vi "initialise.vi"(8 "error in (no error)":errorcluster, 11 "GenericPlugin in":refnum<class "FPGAWrapperRK110512Fiber_Spiral.lvclass">) -> (0 "error out":errorcluster, 3 "GenericPlugin out":refnum<class "FPGAWrapperRK110512Fiber_Spiral.lvclass">)   [LabVIEW 2010, in "FPGAWrapperRK110512Fiber_Spiral.lvclass"]
doc: "The dynamic dispatch-version of this VI initalises the plug-in object by allocating and initalising any dynamic resources need."
uses:
  FPGAWrapperRK110512Fiber_Spiral.lvclass
  GenericFPGAWrapper/GenericFPGAWrapper/GenericFPGAWrapper.lvclass
  <vilib>/rvi/interface/nirviOpenFPGA/nirviOpenFPGA.xnode
  config_data_cluster.ctl
  <vilib>/userDefined/High Color/nirio_resource_hc.ctl
  <vilib>/rvi/interface/nirviMethod/nirviMethod.xnode
  <vilib>/FPGAPlugInAG/Dynamic/niLvFpga_Reset_Dynamic.vi
  <vilib>/rvi/interface/nirviReadWriteControl/nirviReadWriteControl.xnode
  NiFpgaLv.dll
  <vilib>/Utility/error.llb/Error Cluster From Error Code.vi
  <vilib>/rvi/errors/niLvFpgaWhatHappensToTopLevelVI.ctl
  <vilib>/rvi/interface/common/niFpgaNodeNameForErrorReporting.ctl
  <vilib>/rvi/errors/niLvFpgaAdjustHostInterfaceError.vi
  FPGA_VI_Reference.ctl
  FPGA Bitfiles/FPGAWrapperRK120_FPGATarget_FPGASpiral_DEAF4785.lvbitx
  <vilib>/FPGAPlugInAG/PXI-7813R/niLvFpga_Open_PXI-7813R.vi
  <vilib>/rvi/ClientSDK/nirviWhatTheDeviceIsDoing.ctl
  <vilib>/rvi/interface/common/dynamic/niFpgaDynamicAddResources.vi
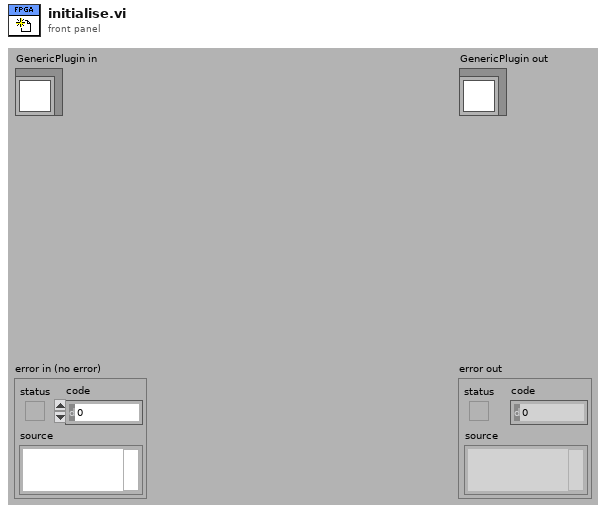
[diagram p1: front panel]
types:
  T1 = typedef "FPGAWrapperRK110512Fiber_Spiral.lvclass/FPGA_VI_Reference.ctl" = refnum<k20>
  T2 = typedef "nirio_resource_hc.ctl" = tag
  T3 = typedef "FPGAWrapperRK110512Fiber_Spiral.lvclass/config_data_cluster.ctl" = cluster{"Hifo box version":i16, "ADC clock phase":u8, "Enable ADC clock":bool, "FPGA Clock":u32}
  T4 = typedef "niFpgaNodeNameForErrorReporting.ctl" = enum16{"Open FPGA VI Reference", "Read/Write Control", "Invoke Method: Abort", "Invoke Method: Acknowledge IRQ", "Invoke Method: Download", "Invoke Method: FIFO.Configure", "Invoke Method: FIFO.Read", "Invoke Method: FIFO.Start", "Invoke Method: FIFO.Stop", "Invoke Method: FIFO.Write", "Invoke Method: Reset", "Invoke Method: Run", "Invoke Method: Wait on IRQ", "Close FPGA VI Reference"}
  T5 = typedef "niLvFpgaWhatHappensToTopLevelVI.ctl" = enum16{"top level VI scripted behind XNode", "top level VI inlined behind XNode"}
  T6 = typedef "nirviWhatTheDeviceIsDoing.ctl" = enum32{"nothing", "something other than LabVIEW FPGA", "FPGA interface", "interactive", "emulation"}
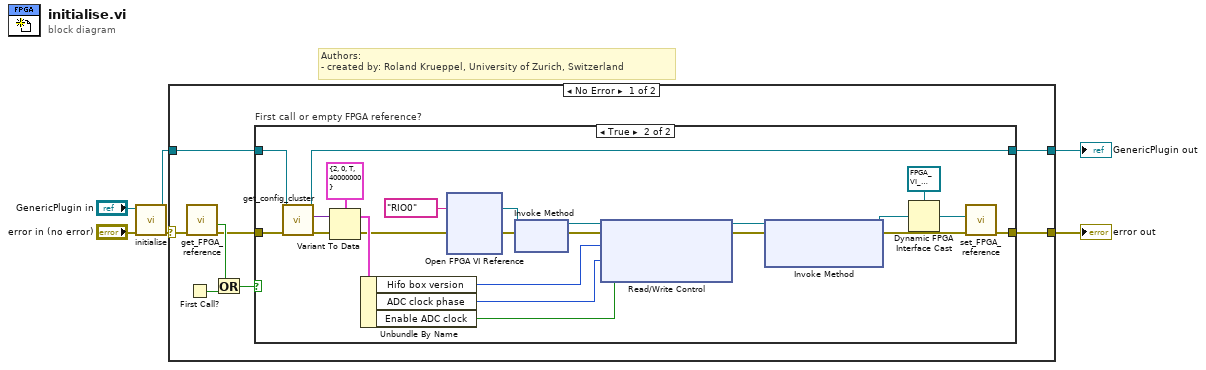
[diagram p0: block diagram]
diagram:
  # "Authors: \n- created by: Roland Krueppel, University of Zurich, Switzerland"
  n1 = call-parent "initialise.vi"("error in (no error)"="error in (no error)", "GenericPlugin in"="GenericPlugin in") -> ("error out"=w4:errorcluster, "GenericPlugin out"=w2:refnum<class "FPGAWrapperRK110512Fiber_Spiral.lvclass">)  [unwired: 8 in]
  n2 = case shown="No Error" w4 {
    selector: w4 -> [w14 w221]
    tunnel: [w7 w221] -> w3
    tunnel: [w10 w222] -> w1
    tunnel: w2 -> [w8 w222]
    frame No Error {
      n3 = First Call?() -> (First Call?: T/F=w13:bool)
      n4 = call "get_FPGA_reference.vi"("error in (no error)"=w14) -> ("error out"=w9:errorcluster, "is empty?"=w12:bool)  [unwired: 8 in, 1 out]
      n5 = Or(x=w12, y=w13) -> (x .or. y?=w11:bool)
      n6 = case "First call or empty FPGA reference?" shown="True" w11 {
        tunnel: [w15 w20] -> w10
        tunnel: w9 -> [w16 w39]
        tunnel: [w16 w22] -> w7
        tunnel: w8 -> [w15 w21]
        frame False {
        }
        frame True {
          n7 = call-dynamic "get_config_cluster.vi"("error in (no error)"=w39, "FPGAWrapperRK120511Fiber_Spiral in"=w21) -> ("error out"=w38:errorcluster, "config cluster (variant)"=w37:variant, "FPGAWrapperRK120511Fiber_Spiral out"=w20:refnum<class "FPGAWrapperRK110512Fiber_Spiral.lvclass">)  [unwired: 7 in]
          n8 = Variant To Data(error in=w38, Variant=w37, type=T3 {"Hifo box version"=2, "ADC clock phase"=0, "Enable ADC clock"=TRUE, "FPGA Clock"=40000000} ("config data")) -> (error out=w34:errorcluster, data=w35:T3)
          n9 = Unbundle By Name(w35) -> ("Hifo box version"=w28:i16, "ADC clock phase"=w27:u8, "Enable ADC clock"=w26:bool)
          n10 = xnode "Open FPGA VI Reference"("error in"=w34, "resource name"=T2 "RIO0") -> ("FPGA VI Reference Out"=w31:refnum<k20>, "error out"=w32:errorcluster)
          n11 = xnode "Invoke Method"("FPGA VI Reference In"=w31, "error in"=w32) -> ("FPGA VI Reference Out"=w29:refnum<k20>, "error out"=w30:errorcluster)
          n12 = xnode "Read/Write Control"("FPGA VI Reference In"=w29, "error in"=w30, "converter box version"=w28, "ADC clock phase"=w27, "Enable ADC clock?"=w26) -> ("FPGA VI Reference Out"=w25:refnum<k20>, "error out"=w24:errorcluster)
          n13 = xnode "Invoke Method"("FPGA VI Reference In"=w25, "error in"=w24) -> ("FPGA VI Reference Out"=w19:refnum<k20>, "error out"=w23:errorcluster)  [unwired: 1 in]
          n14 = Dynamic FPGA Interface Cast(Session In=T1 refnum ("FPGA VI Reference"), Type=w19) -> (Session Out=w17:T1)
          n15 = call "set_FPGA_reference.vi"("error in (no error)"=w23, "FPGA VI Reference"=w17) -> ("error out"=w22:errorcluster)  [unwired: 9 in]
        }
      }
    }
    frame Error {
    }
  }
  "error out" <- w3
  "GenericPlugin out" <- w1
